vi "Create Execution Events.vi"() -> (3 "Execution Events":T1)   [LabVIEW 2022 SP3, in "FlexBlocks Support.lvlib"]
uses:
  FlexBlocks Support.lvlib
  Block Phase.ctl
  Block State.ctl
  Block Status.ctl
  Block Status with Error.ctl
  Block Command.ctl
  Worker Block.ctl
  Worker Registration.ctl
  Execution Events.ctl
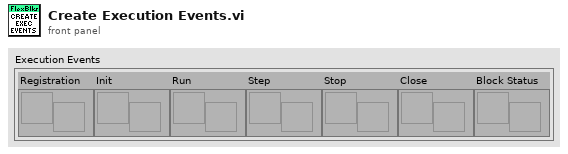
[diagram p1: front panel]
types:
  T1 = typedef "FlexBlocks Support.lvlib/Execution Events.ctl" = cluster{"Registration":refnum<user-event>, "Init":refnum<user-event>, "Run":refnum<user-event>, "Step":refnum<user-event>, "Stop":refnum<user-event>, "Close":refnum<user-event>, "Block Status":refnum<user-event>}
  T2 = typedef "FlexBlocks Support.lvlib/Block Status with Error.ctl" = cluster{"Block Status":T3, "Error":errorcluster}
  T3 = typedef "FlexBlocks Support.lvlib/Block Status.ctl" = cluster{"State":T4, "Runs":u32, "i":i32, "Init":bool, "Started":bool, "Closing":bool, "Phase":T5, "Worker":string}
  T4 = typedef "FlexBlocks Support.lvlib/Block State.ctl" = enum16{"Idle", "Init", "Start", "Run", "Stop", "Close"}
  T5 = typedef "FlexBlocks Support.lvlib/Block Phase.ctl" = enum16{"N/A", "Read", "Work", "Write"}
  T6 = typedef "FlexBlocks Support.lvlib/Worker Registration.ctl" = cluster{"Worker":string, "Response":refnum<notifier>}
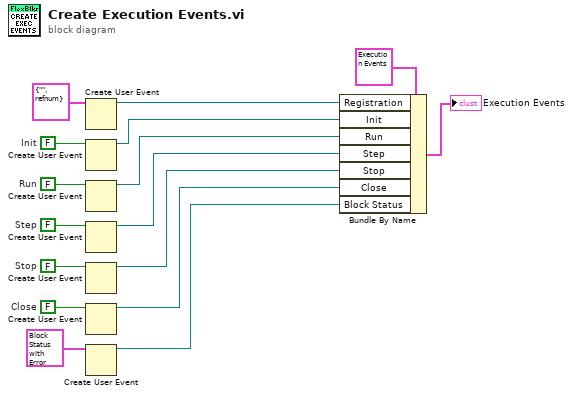
[diagram p0: block diagram]
diagram:
  w11 = FALSE  # Close
  w12 = FALSE  # Stop
  w13 = FALSE  # Step
  w14 = FALSE  # Run
  w15 = FALSE  # Init
  n1 = Create User Event(user event datatype=T6 {"Worker"="", "Response"=refnum} ("Worker Registration")) -> (user event=w9:refnum<user-event>)  [unwired: 1 in, 1 out]
  n2 = Create User Event(user event datatype=w15) -> (user event=w8:refnum<user-event>)  [unwired: 1 in, 1 out]
  n3 = Create User Event(user event datatype=w14) -> (user event=w7:refnum<user-event>)  [unwired: 1 in, 1 out]
  n4 = Create User Event(user event datatype=w13) -> (user event=w6:refnum<user-event>)  [unwired: 1 in, 1 out]
  n5 = Create User Event(user event datatype=w12) -> (user event=w5:refnum<user-event>)  [unwired: 1 in, 1 out]
  n6 = Create User Event(user event datatype=w11) -> (user event=w4:refnum<user-event>)  [unwired: 1 in, 1 out]
  n7 = Create User Event(user event datatype=T2 {"Block Status"={"State"=enum."Init", "Runs"=0, "i"=0, "Init"=FALSE, "Started"=FALSE, "Closing"=FALSE, "Phase"=enum."N/A", "Worker"=""}, "Error"={"status"=FALSE, "code"=0, "source"=""}} ("Block Status with Error")) -> (user event=w1:refnum<user-event>)  [unwired: 1 in, 1 out]
  n8 = Bundle By Name(cluster=T1 {"Registration"=refnum, "Init"=refnum, "Run"=refnum, "Step"=refnum, "Stop"=refnum, "Close"=refnum, "Block Status"=refnum} ("Execution Events"), "Registration"=w9, "Init"=w8, "Run"=w7, "Step"=w6, "Stop"=w5, "Close"=w4, "Block Status"=w1) -> (→"Execution Events":T1)
